vi "XY Graph Replace Multiplots with Names.vi"(0 "XYGraph in":T3, 1 "Array of Scales (Default)":cluster{"X Scale":u32, "Y Scale":u32}[](array[cluster]), 2 "Plots Interpolation (Previous Plot's Style)":T2[](array[typedef]), 3 "Replaced Plots Indices (last)":i32[](array[numeric]), 5 "Array of Plots":cluster{"X Array":dbl[], "Y Array":dbl[]}[](array[cluster]), 7 "Plots Metadata":variant[](array[variant]), 9 "Array of Plot Names (\"Plot\")":string[](array[string]), 11 "error in (no error)":errorcluster, 12 "Make Visible (T)":bool=TRUE, 13 "Plot Colors (Default)":u32[](array[colorbox]), 14 "Point Style (Dot)":T1=enum."Dot") -> (4 "XY Graph Caption":string, 6 "Total Number of Plots":i32, 8 "Number of Plots Added":i32, 10 "Added Plot Names":string[](array[string]), 15 "error out":errorcluster)   [LabVIEW 2021, in "XY Graph Add-Ons.lvlib"]
uses:
  XY Graph Add-Ons.lvlib
  XY Graph Refnum.ctl
  LabVIEW Plot Interpolation.ctl
  Plot Point Style.ctl
  XY Graph Get Plots Metadata.vi
  XY Graph Set Plots Metadata.vi
  Strings/Strings.lvlib
  Graphs.lvlib
  Error/Error.lvlib
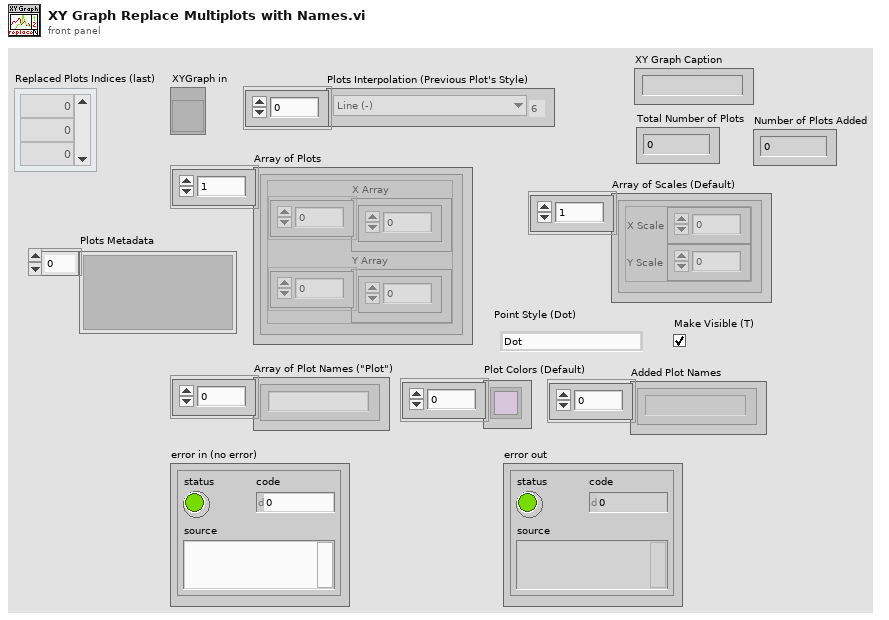
[diagram p1: front panel]
types:
  T1 = typedef "Graphs.lvlib/Plot Point Style.ctl" = enum16{"not defined", "None", "Empty Circle", "Filled Circle", "Thick Circle", "Dotted Circle", "Empty Square", "Filled Square", "Thick Square", "Dotted Square", "Small Filled Square", "Dot", "Cross", "Tiny Cross", "Large X", "Small x", "Diamond", "Small Empty Square"}
  T2 = typedef "Graphs.lvlib/LabVIEW Plot Interpolation.ctl" = enum16{"Point (.)", "Stepwise Right (--.)", "Line + Point (\\. /)", "Stepwise Left (.--)", "Stepwise Centered (-.-)", "Stepwise Vertical (|.|)", "Line (-)", "Use Previous Plot's Style"}
  T3 = typedef "XY Graph Add-Ons.lvlib/XY Graph Refnum.ctl" = refnum<vi>
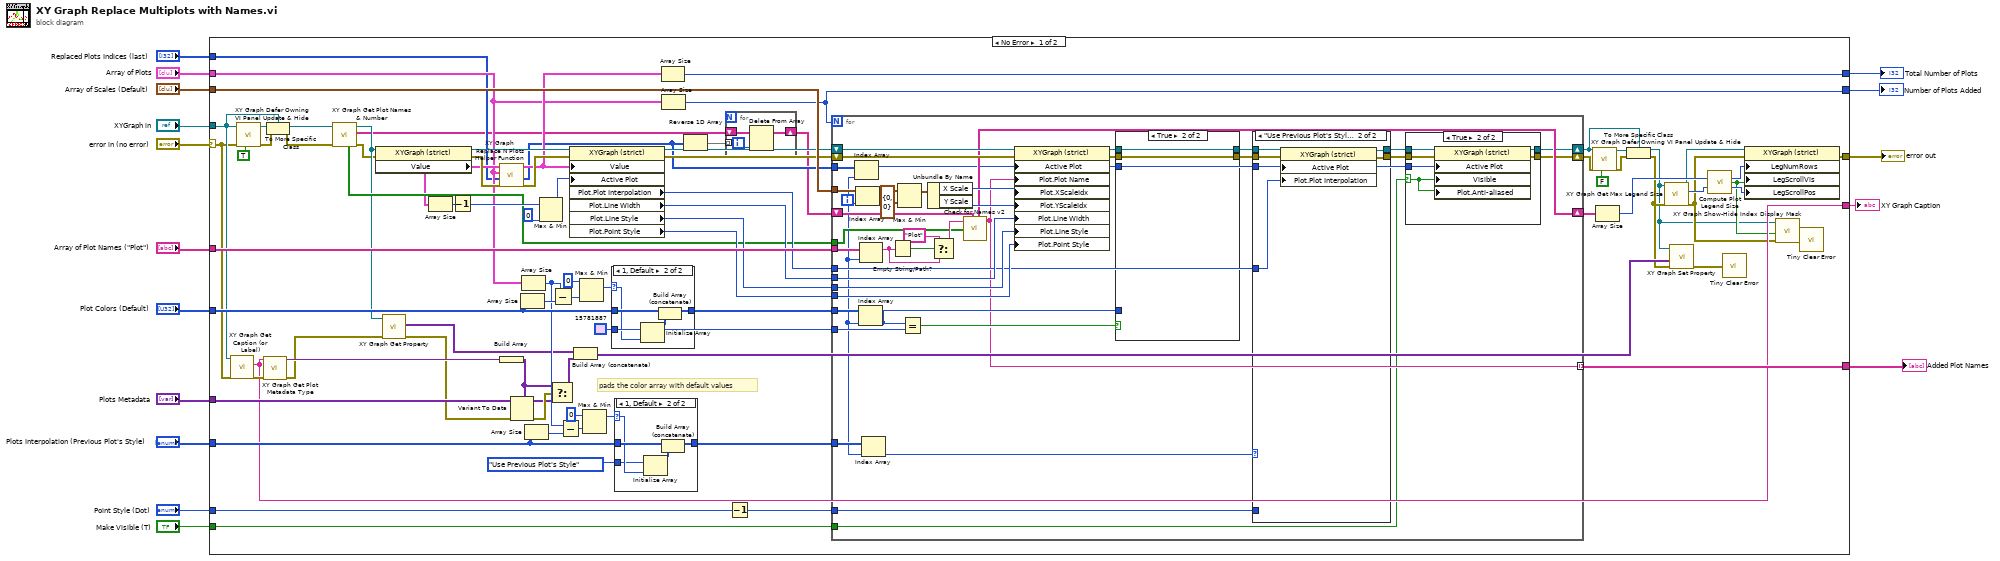
[diagram p0: block diagram]
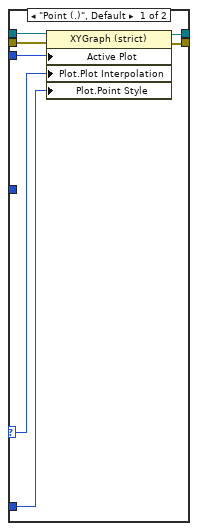
[diagram p3: hidden frame]
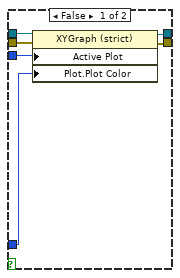
[diagram p4: hidden frame]
diagram:
  n1 = case shown="No Error" "error in (no error)" {
    selector: "error in (no error)" -> [w36 w185]
    tunnel: "XYGraph in" -> [w46 _]
    tunnel: "Array of Plot Names (\"Plot\")" -> [w98 _]
    tunnel: "Array of Scales (Default)" -> [w97 _]
    tunnel: [w91 _] -> w12
    tunnel: "Array of Plots" -> [w22 _]
    tunnel: "Plot Colors (Default)" -> [w87 _]
    tunnel: "Plots Interpolation (Previous Plot's Style)" -> [w84 _]
    tunnel: [w73 w185] -> w8
    tunnel: [w72 _] -> w7
    tunnel: "Point Style (Dot)" -> [w71 _]
    tunnel: "Make Visible (T)" -> [w69 _]
    tunnel: [w68 _] -> w4
    tunnel: [w34 _] -> w3
    tunnel: "Plots Metadata" -> [w44 _]
    tunnel: "Replaced Plots Indices (last)" -> [w21 _]
    frame No Error {
      w85 = u32 15781887 ("Plot Color (Default)")
      # "pads the color array with default values"
      n2 = call "XY Graph Get Caption (or Label).vi"("error in (no error)"=w36, "XY Graph in"=w46) -> ("error out"=w35:errorcluster, "Caption (or Label) Text"=w34:string)  [unwired: 7 in, 1 out]
      n3 = call "XY Graph Defer Owning VI Panel Update & Hide.vi"("Defer Owning Panel Update"=TRUE, "error in (no error)"=w36, "XY Graph Refnum in"=w46) -> ("error out"=w59:errorcluster, "XY Graph Refnum out"=w62:refnum<vi>)  [unwired: 7 in]
      n4 = call "XY Graph Get Plot Metadata Type.vi"("Error In"=w35, "Graph Label"=w34) -> ("Error Out"=w39:errorcluster, "Plot Metadata Type"=w45:variant)  [unwired: 7 in, 1 out]
      n5 = To More Specific Class(target class=w46, reference=w62, error in=w59) -> (specific class reference=w60:T3, error out=w58:errorcluster)
      n6 = call "XY Graph Get Plot Names & Number.vi"("error in (no error)"=w58, "XYGraph in"=w60) -> ("error out"=w27:errorcluster, "Plot Names"=w20:string[], "XYGraph out"=w28:T3, "Empty Plots?"=w61:bool[])  [unwired: 4 in, 2 out]
      n7 = property class="XYGraph (strict)"(reference=w28, error in=w27) -> (reference out=w99:T3, error out=w26:errorcluster, "Value"=w24:cluster{"X Array":dbl[], "Y Array":dbl[]}[])
      n8 = call-poly "XY Graph Get Property.vi"("Error In"=w39, "XYGraph Ref"=w28) -> ("Error Out"=w38:errorcluster, "Plot Metadata"=w49:variant[])  [unwired: 6 in, 2 out]
      n9 = Array Size(array=w24) -> (size(s)=w29:i32)
      n10 = Decrement(x=w29) -> (x-1=w96:i32)
      n11 = call "XY Graph Replace N Plots Helper Function.vi"("error in (no error)"=w26, "Replaced Plots Indices (last plots)"=w21, "Array of Plots"=w22, "Current Plots"=w24) -> ("error out"=w25:errorcluster, "Replaced Plots Indices"=w19:i32[], "New Plots"=w23:cluster{"X Array":dbl[], "Y Array":dbl[]}[])  [unwired: 5 in]
      n12 = Build Array(w45) -> (w41:variant[])
      n13 = Variant To Data(error in=w38, type=w41, Variant=w44) -> (data=w42:variant[], error out=w43:errorcluster)
      n14 = Array Size(array=w87) -> (size(s)=w82:i32)
      n15 = Array Size(array=w22) -> (size(s)=w76:i32)
      n16 = Array Size(array=w84) -> (size(s)=w83:i32)
      n17 = Max & Min(x=w96, y=0) -> (max(x,y)=w75:i32)  [unwired: 1 out]
      n18 = Select(t=w41, s=w43, f=w42) -> (s? t:f=w40:variant[])
      n19 = Subtract(x=w76, y=w82) -> (x-y=w90:i32)
      n20 = Subtract(x=w76, y=w83) -> (x-y=w81:i32)
      n21 = property class="XYGraph (strict)"(reference=w99, error in=w25, "Value"=w23, "Active Plot"=w75) -> (reference out=w67:T3, error out=w66:errorcluster, "Plot.Plot Interpolation"=w95:u8, "Plot.Line Width"=w94:u8, "Plot.Line Style"=w93:u8, "Plot.Point Style"=w92:u8)
      n22 = Build Array (concatenate)(w49, w40) -> (w48:variant[])
      n23 = Max & Min(x=0, y=w90) -> (max(x,y)=w88:i32)  [unwired: 1 out]
      n24 = Max & Min(x=0, y=w81) -> (max(x,y)=w79:i32)  [unwired: 1 out]
      n25 = case shown="1, Default" w88 {
        selector: w88 -> [_ w182]
        tunnel: w87 -> [w179 w184]
        tunnel: [w179 w183] -> w86
        tunnel: w85 -> [_ w180]
        frame 0 {
        }
        frame 1, Default {
          n26 = Initialize Array(w180, w182) -> (w181:u32[])
          n27 = Build Array (concatenate)(w184, w181) -> (w183:u32[])
        }
      }
      n28 = case shown="1, Default" w79 {
        selector: w79 -> [_ w176]
        tunnel: w84 -> [w173 w178]
        tunnel: [w173 w177] -> w78
        tunnel: LabVIEW_Plot_Interpolation."Use Previous Plot's Style" ("Plot Interpolation") -> [_ w174]
        frame 0 {
        }
        frame 1, Default {
          n29 = Initialize Array(w174, w176) -> (w175:T2[])
          n30 = Build Array (concatenate)(w178, w175) -> (w177:T2[])
        }
      }
      n31 = Array Size(array=w23) -> (size(s)=w72:i32)
      n32 = Array Size(array=w22) -> (size(s)=w68:i32)
      n33 = Reverse 1D Array(array=w19) -> (reversed array=w18:i32[])
      n34 = for {
        shift-right: [w101] -> w17
        shift-left: w20 -> [w103]
        tunnel: w18 -> [w102] mode=indexing
        n35 = Delete From Array(array=w103, index=w102) -> (array with subset deleted=w101:string[])  [unwired: 1 in, 1 out]
      }
      n36 = Decrement(x=w71) -> (x-1=w70:T1)
      n37 = for {
        N: w68 -> [_]
        tunnel: w98 -> [w141]
        shift-right: [w110] -> w65
        shift-left: w66 -> [w142]
        shift-right: [w113] -> w51
        shift-left: w67 -> [w143]
        shift-right: [w116] -> w100
        shift-left: w17 -> [w117]
        tunnel: w97 -> [w140]
        tunnel: w95 -> [w119]
        tunnel: w94 -> [w133]
        tunnel: w93 -> [w132]
        tunnel: w92 -> [w131]
        tunnel: [w114] -> w91 mode=indexing
        tunnel: w86 -> [w130]
        tunnel: w85 -> [w129]
        tunnel: w78 -> [w121]
        tunnel: w70 -> [w118]
        tunnel: w69 -> [w112]
        tunnel: w61 -> [w107]
        tunnel: w19 -> [w106]
        i -> [w105]
        n38 = Index Array(array=w106, index=w105) -> (element=w104:i32)
        n39 = Index Array(array=w140, index=w105) -> (element=w139:cluster{"X Scale":u32, "Y Scale":u32})
        n40 = Index Array(array=w130, index=w105) -> (element=w125:u32)
        n41 = Index Array(array=w141, index=w105) -> (element=w135:string)
        n42 = Index Array(array=w121, index=w105) -> (element=w120:T2)
        n43 = Empty String/Path?(string/path=w135) -> (empty?=w136:bool)
        n44 = Max & Min(x=w139, y=cluster{"X Scale":u32, "Y Scale":u32} {"X Scale"=0, "Y Scale"=0}) -> (max(x,y)=w109:cluster{"X Scale":u32, "Y Scale":u32})  [unwired: 1 out]
        n45 = Equal?(x=w125, y=w129) -> (x = y?=w128:bool)
        n46 = Unbundle By Name(w109) -> ("X Scale"=w138:u32, "Y Scale"=w137:u32)
        n47 = Select(t="Plot", s=w136, f=w135) -> (s? t:f=w115:string)
        n48 = call "Check for Names v2.vi"("New Name"=w115, "Name List"=w117, "Empty Plots?"=w107) -> ("New Name List"=w116:string[], "New Name"=w114:string)  [unwired: 3 in, 2 out]
        n49 = property class="XYGraph (strict)"(reference=w143, error in=w142, "Active Plot"=w104, "Plot.Plot Name"=w114, "Plot.XScaleIdx"=w138, "Plot.YScaleIdx"=w137, "Plot.Line Width"=w133, "Plot.Line Style"=w132, "Plot.Point Style"=w131) -> (reference out=w127:T3, error out=w126:errorcluster)
        n50 = case shown="True" w128 {
          tunnel: w127 -> [w170 w172]
          tunnel: [w169 w172] -> w124
          tunnel: w126 -> [w168 w171]
          tunnel: [w167 w171] -> w123
          tunnel: w125 -> [w166 _]
          tunnel: w104 -> [w165 _]
          frame False {
            n51 = property class="XYGraph (strict)"(reference=w170, error in=w168, "Active Plot"=w165, "Plot.Plot Color"=w166) -> (reference out=w169:T3, error out=w167:errorcluster)
          }
          frame True {
          }
        }
        n52 = case shown="\"Use Previous Plot's Style\"" w120 {
          selector: w120 -> [w153 _]
          tunnel: w124 -> [w158 w164]
          tunnel: [w157 w163] -> w122
          tunnel: w123 -> [w156 w162]
          tunnel: [w155 w161] -> w111
          tunnel: w104 -> [w154 w160]
          tunnel: w119 -> [_ w159]
          tunnel: w118 -> [w152 _]
          frame "Point (.)", Default {
            n53 = property class="XYGraph (strict)"(reference=w158, error in=w156, "Active Plot"=w154, "Plot.Plot Interpolation"=w153, "Plot.Point Style"=w152) -> (reference out=w157:T3, error out=w155:errorcluster)
          }
          frame "Use Previous Plot's Style" {
            n54 = property class="XYGraph (strict)"(reference=w164, error in=w162, "Active Plot"=w160, "Plot.Plot Interpolation"=w159) -> (reference out=w163:T3, error out=w161:errorcluster)
          }
        }
        n55 = case shown="True" w112 {
          selector: w112 -> [_ w146]
          tunnel: w122 -> [w145 w151]
          tunnel: [w145 w150] -> w113
          tunnel: w111 -> [w144 w149]
          tunnel: [w144 w148] -> w110
          tunnel: w104 -> [_ w147]
          frame False {
          }
          frame True {
            n56 = property class="XYGraph (strict)"(reference=w151, error in=w149, "Active Plot"=w147, "Visible"=w146, "Plot.Anti-aliased"=w146) -> (reference out=w150:T3, error out=w148:errorcluster)
          }
        }
      }
      n57 = call "XY Graph Defer Owning VI Panel Update & Hide.vi"("Defer Owning Panel Update"=FALSE, "error in (no error)"=w65, "XY Graph Refnum in"=w51) -> ("error out"=w53:errorcluster, "XY Graph Refnum out"=w52:refnum<vi>)  [unwired: 7 in]
      n58 = Array Size(array=w100) -> (size(s)=w56:i32)
      n59 = To More Specific Class(target class=w51, reference=w52, error in=w53) -> (specific class reference=w30:T3, error out=w47:errorcluster)
      n60 = call "XY Graph Get Max Legend Size.vi"("Error In"=w47, "XYGraph Refnum"=w30) -> ("Error Out"=w32:errorcluster, "Max Legend Size"=w57:i32, "XYGraph Refnum"=w50:T3)  [unwired: 6 in, 1 out]
      n61 = call-poly "XY Graph Set Property.vi"("error in (no error)"=w47, "Plots Metadata"=w48, "XY Graph Refnum"=w30) -> ("error out"=w37:errorcluster)  [unwired: 7 in, 1 out]
      n62 = call "Compute Plot Legend Size.vi"("# Plots"=w56, "Max Legend Size"=w57) -> ("LegNumRows"=w55:u32, "LegScrollVis"=w31:bool, "LegScrollPos"=w54:u32)  [unwired: 11 in]
      n63 = call "Tiny Clear Error.vi"("Error In"=w37) -> ()  [unwired: 8 in, 1 out]
      n64 = property class="XYGraph (strict)"(reference=w50, error in=w32, "LegNumRows"=w55, "LegScrollVis"=w31, "LegScrollPos"=w54) -> (error out=w73:errorcluster)  [unwired: 1 out]
      n65 = call "XY Graph Show-Hide Index Display Mask.vi"("error in (no error)"=w32, "Show(T)/Hide(F)"=w31, "XYGraph Ref"=w30) -> ("error out"=w33:errorcluster)  [unwired: 7 in, 1 out]
      n66 = call "Tiny Clear Error.vi"("Error In"=w33) -> ()  [unwired: 8 in, 1 out]
    }
    frame Error {
    }
  }
  "error out" <- w8
  "Added Plot Names" <- w12
  "Total Number of Plots" <- w7
  "Number of Plots Added" <- w4
  "XY Graph Caption" <- w3
